vi "Register gRPC Methods.vi"(8 "error in (no error)":errorcluster, 11 "Template Server in":refnum<class "NiDAQmx.lvclass">) -> (0 "error out":errorcluster, 3 "Template Server out":refnum<class "NiDAQmx.lvclass">)   [LabVIEW 2021, in "NI DAQmx_server.lvlib" / "NiDAQmx.lvclass"]
uses:
  NiDAQmx.lvclass
  typeDefs/Server Internal UEs.ctl
  typeDefs/Server Internal Message.ctl
  typeDefs/Server gRPC UEs.ctl
  <vilib>/gRPC/LabVIEW gRPC Library/Server API/typeDefs/gRPCId Cluster.ctl
  <vilib>/gRPC/LabVIEW gRPC Library/Shared/grpcId.ctl
  NiDAQmx.lvclass/NiDAQmx.ctl
  <vilib>/gRPC/LabVIEW gRPC Library/grpc-lvsupport-release.lvlib
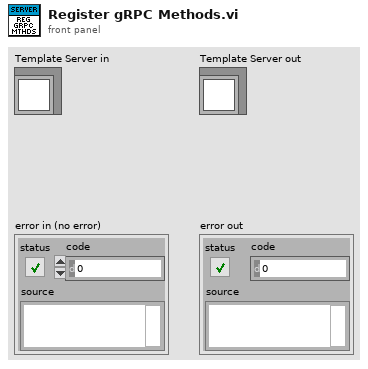
[diagram p1: front panel]
types:
  T1 = typedef "NI DAQmx_server.lvlib/NiDAQmx.lvclass/Server gRPC UEs.ctl" = cluster{"NiDAQmx CreateTask gRPC UE":refnum<user-event>, "NiDAQmx CreateDOChan gRPC UE":refnum<user-event>, "NiDAQmx CreateCIFreqChan gRPC UE":refnum<user-event>, "NiDAQmx WriteDigitalLines gRPC UE":refnum<user-event>, "NiDAQmx ReadCounterScalarF64 gRPC UE":refnum<user-event>, "NiDAQmx CfgImplicitTiming gRPC UE":refnum<user-event>, "NiDAQmx StartTask gRPC UE":refnum<user-event>, "NiDAQmx StopTask gRPC UE":refnum<user-event>, "NiDAQmx ClearTask gRPC UE":refnum<user-event>, "NiDAQmx GetTaskAttributeString gRPC UE":refnum<user-event>, "NiDAQmx GetChanAttributeString gRPC UE":refnum<user-event>, "NiDAQmx GetChanAttributeDouble gRPC UE":refnum<user-event>, "NiDAQmx SetChanAttributeString gRPC UE":refnum<user-event>, "NiDAQmx SetChanAttributeDouble gRPC UE":refnum<user-event>}
  T2 = typedef "NI DAQmx_server.lvlib/NiDAQmx.lvclass/Server Internal UEs.ctl" = cluster{"NiDAQmx CreateTask Internal UE":refnum<user-event>, "NiDAQmx CreateDOChan Internal UE":refnum<user-event>, "NiDAQmx CreateCIFreqChan Internal UE":refnum<user-event>, "NiDAQmx WriteDigitalLines Internal UE":refnum<user-event>, "NiDAQmx ReadCounterScalarF64 Internal UE":refnum<user-event>, "NiDAQmx CfgImplicitTiming Internal UE":refnum<user-event>, "NiDAQmx StartTask Internal UE":refnum<user-event>, "NiDAQmx StopTask Internal UE":refnum<user-event>, "NiDAQmx ClearTask Internal UE":refnum<user-event>, "NiDAQmx GetTaskAttributeString Internal UE":refnum<user-event>, "NiDAQmx GetChanAttributeString Internal UE":refnum<user-event>, "NiDAQmx GetChanAttributeDouble Internal UE":refnum<user-event>, "NiDAQmx SetChanAttributeString Internal UE":refnum<user-event>, "NiDAQmx SetChanAttributeDouble Internal UE":refnum<user-event>}
  T3 = typedef "grpc-lvsupport-release.lvlib/grpcId.ctl" = u64
  T4 = typedef "NI DAQmx_server.lvlib/NiDAQmx.lvclass/Server Internal Message UE.ctl" = refnum<user-event>
  T5 = typedef "grpc-lvsupport-release.lvlib/gRPCId Cluster UE.ctl" = refnum<user-event>
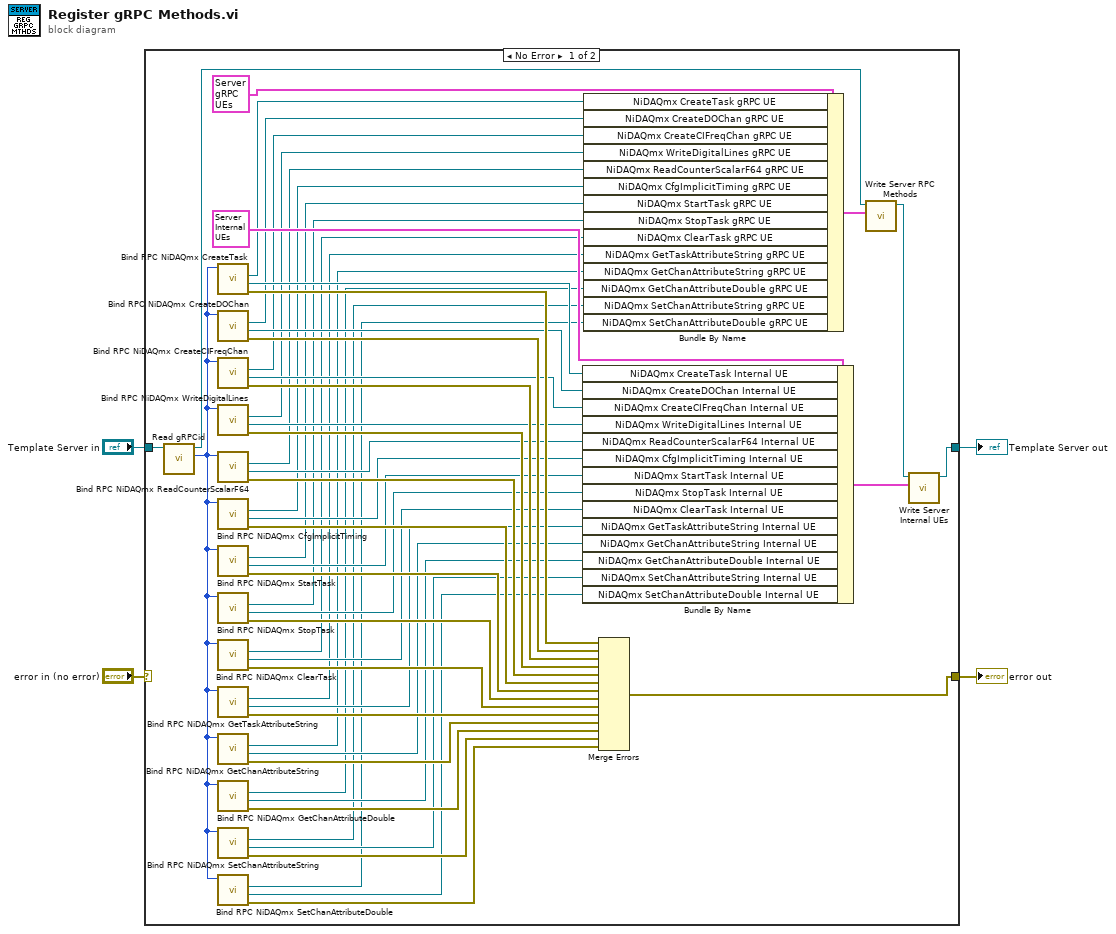
[diagram p0: block diagram]
diagram:
  n1 = case shown="No Error" "error in (no error)" {
    selector: "error in (no error)" -> [_ w57]
    tunnel: "Template Server in" -> [w48 w58]
    tunnel: [w56 w57] -> w3
    tunnel: [w55 w58] -> w2
    frame No Error {
      n2 = call-dynamic "Read gRPCid.vi"("iService in"=w48) -> ("gRPCid"=w47:T3, "iService out"=w49:refnum<class "NiDAQmx.lvclass">)  [unwired: 8 in, 1 out]
      n3 = call "Bind RPC NiDAQmx CreateTask.vi"("gRPCid server in"=w47) -> ("error out"=w46:errorcluster, "NiDAQmx CreateTask Internal UE"=w44:T4, "NiDAQmx CreateTask gRPC UE"=w45:T5)  [unwired: 7 in, 1 out]
      n4 = call "Bind RPC NiDAQmx CreateDOChan.vi"("gRPCid server in"=w47) -> ("error out"=w43:errorcluster, "NiDAQmx CreateDOChan Internal UE"=w41:T4, "NiDAQmx CreateDOChan gRPC UE"=w42:T5)  [unwired: 7 in, 1 out]
      n5 = call "Bind RPC NiDAQmx CreateCIFreqChan.vi"("gRPCid server in"=w47) -> ("error out"=w40:errorcluster, "NiDAQmx CreateCIFreqChan Internal UE"=w38:T4, "NiDAQmx CreateCIFreqChan gRPC UE"=w39:T5)  [unwired: 7 in, 1 out]
      n6 = call "Bind RPC NiDAQmx WriteDigitalLines.vi"("gRPCid server in"=w47) -> ("error out"=w37:errorcluster, "NiDAQmx WriteDigitalLines Internal UE"=w35:T4, "NiDAQmx WriteDigitalLines gRPC UE"=w36:T5)  [unwired: 7 in, 1 out]
      n7 = call "Bind RPC NiDAQmx ReadCounterScalarF64.vi"("gRPCid server in"=w47) -> ("error out"=w34:errorcluster, "NiDAQmx ReadCounterScalarF64 Internal UE"=w32:T4, "NiDAQmx ReadCounterScalarF64 gRPC UE"=w33:T5)  [unwired: 7 in, 1 out]
      n8 = call "Bind RPC NiDAQmx CfgImplicitTiming.vi"("gRPCid server in"=w47) -> ("error out"=w31:errorcluster, "NiDAQmx CfgImplicitTiming Internal UE"=w29:T4, "NiDAQmx CfgImplicitTiming gRPC UE"=w30:T5)  [unwired: 7 in, 1 out]
      n9 = call "Bind RPC NiDAQmx StartTask.vi"("gRPCid server in"=w47) -> ("error out"=w28:errorcluster, "NiDAQmx StartTask Internal UE"=w26:T4, "NiDAQmx StartTask gRPC UE"=w27:T5)  [unwired: 7 in, 1 out]
      n10 = call "Bind RPC NiDAQmx StopTask.vi"("gRPCid server in"=w47) -> ("error out"=w25:errorcluster, "NiDAQmx StopTask Internal UE"=w23:T4, "NiDAQmx StopTask gRPC UE"=w24:T5)  [unwired: 7 in, 1 out]
      n11 = call "Bind RPC NiDAQmx ClearTask.vi"("gRPCid server in"=w47) -> ("error out"=w22:errorcluster, "NiDAQmx ClearTask Internal UE"=w20:T4, "NiDAQmx ClearTask gRPC UE"=w21:T5)  [unwired: 7 in, 1 out]
      n12 = call "Bind RPC NiDAQmx GetTaskAttributeString.vi"("gRPCid server in"=w47) -> ("error out"=w19:errorcluster, "NiDAQmx GetTaskAttributeString Internal UE"=w17:T4, "NiDAQmx GetTaskAttributeString gRPC UE"=w18:T5)  [unwired: 7 in, 1 out]
      n13 = call "Bind RPC NiDAQmx GetChanAttributeString.vi"("gRPCid server in"=w47) -> ("error out"=w16:errorcluster, "NiDAQmx GetChanAttributeString Internal UE"=w14:T4, "NiDAQmx GetChanAttributeString gRPC UE"=w15:T5)  [unwired: 7 in, 1 out]
      n14 = call "Bind RPC NiDAQmx GetChanAttributeDouble.vi"("gRPCid server in"=w47) -> ("error out"=w13:errorcluster, "NiDAQmx GetChanAttributeDouble Internal UE"=w11:T4, "NiDAQmx GetChanAttributeDouble gRPC UE"=w12:T5)  [unwired: 7 in, 1 out]
      n15 = call "Bind RPC NiDAQmx SetChanAttributeString.vi"("gRPCid server in"=w47) -> ("error out"=w10:errorcluster, "NiDAQmx SetChanAttributeString Internal UE"=w8:T4, "NiDAQmx SetChanAttributeString gRPC UE"=w9:T5)  [unwired: 7 in, 1 out]
      n16 = call "Bind RPC NiDAQmx SetChanAttributeDouble.vi"("gRPCid server in"=w47) -> ("error out"=w7:errorcluster, "NiDAQmx SetChanAttributeDouble Internal UE"=w5:T4, "NiDAQmx SetChanAttributeDouble gRPC UE"=w6:T5)  [unwired: 7 in, 1 out]
      n17 = Bundle By Name ("Bundle Internal UEs")(cluster=T2 {"NiDAQmx CreateTask Internal UE"=refnum, "NiDAQmx CreateDOChan Internal UE"=refnum, "NiDAQmx CreateCIFreqChan Internal UE"=refnum, "NiDAQmx WriteDigitalLines Internal UE"=refnum, "NiDAQmx ReadCounterScalarF64 Internal UE"=refnum, "NiDAQmx CfgImplicitTiming Internal UE"=refnum, "NiDAQmx StartTask Internal UE"=refnum, "NiDAQmx StopTask Internal UE"=refnum, "NiDAQmx ClearTask Internal UE"=refnum, "NiDAQmx GetTaskAttributeString Internal UE"=refnum, "NiDAQmx GetChanAttributeString Internal UE"=refnum, "NiDAQmx GetChanAttributeDouble Internal UE"=refnum, "NiDAQmx SetChanAttributeString Internal UE"=refnum, "NiDAQmx SetChanAttributeDouble Internal UE"=refnum} ("Server Internal UEs"), "NiDAQmx CreateTask Internal UE"=w44, "NiDAQmx CreateDOChan Internal UE"=w41, "NiDAQmx CreateCIFreqChan Internal UE"=w38, "NiDAQmx WriteDigitalLines Internal UE"=w35, "NiDAQmx ReadCounterScalarF64 Internal UE"=w32, "NiDAQmx CfgImplicitTiming Internal UE"=w29, "NiDAQmx StartTask Internal UE"=w26, "NiDAQmx StopTask Internal UE"=w23, "NiDAQmx ClearTask Internal UE"=w20, "NiDAQmx GetTaskAttributeString Internal UE"=w17, "NiDAQmx GetChanAttributeString Internal UE"=w14, "NiDAQmx GetChanAttributeDouble Internal UE"=w11, "NiDAQmx SetChanAttributeString Internal UE"=w8, "NiDAQmx SetChanAttributeDouble Internal UE"=w5) -> (w54:T2)
      n18 = Bundle By Name ("Bundle gRPC UEs")(cluster=T1 {"NiDAQmx CreateTask gRPC UE"=refnum, "NiDAQmx CreateDOChan gRPC UE"=refnum, "NiDAQmx CreateCIFreqChan gRPC UE"=refnum, "NiDAQmx WriteDigitalLines gRPC UE"=refnum, "NiDAQmx ReadCounterScalarF64 gRPC UE"=refnum, "NiDAQmx CfgImplicitTiming gRPC UE"=refnum, "NiDAQmx StartTask gRPC UE"=refnum, "NiDAQmx StopTask gRPC UE"=refnum, "NiDAQmx ClearTask gRPC UE"=refnum, "NiDAQmx GetTaskAttributeString gRPC UE"=refnum, "NiDAQmx GetChanAttributeString gRPC UE"=refnum, "NiDAQmx GetChanAttributeDouble gRPC UE"=refnum, "NiDAQmx SetChanAttributeString gRPC UE"=refnum, "NiDAQmx SetChanAttributeDouble gRPC UE"=refnum} ("gRPC Server Method Events"), "NiDAQmx CreateTask gRPC UE"=w45, "NiDAQmx CreateDOChan gRPC UE"=w42, "NiDAQmx CreateCIFreqChan gRPC UE"=w39, "NiDAQmx WriteDigitalLines gRPC UE"=w36, "NiDAQmx ReadCounterScalarF64 gRPC UE"=w33, "NiDAQmx CfgImplicitTiming gRPC UE"=w30, "NiDAQmx StartTask gRPC UE"=w27, "NiDAQmx StopTask gRPC UE"=w24, "NiDAQmx ClearTask gRPC UE"=w21, "NiDAQmx GetTaskAttributeString gRPC UE"=w18, "NiDAQmx GetChanAttributeString gRPC UE"=w15, "NiDAQmx GetChanAttributeDouble gRPC UE"=w12, "NiDAQmx SetChanAttributeString gRPC UE"=w9, "NiDAQmx SetChanAttributeDouble gRPC UE"=w6) -> (w51:T1)
      n19 = Merge Errors(w46, w43, w40, w37, w34, w31, w28, w25, w22, w19, w16, w13, w10, w7) -> (w56:errorcluster)
      n20 = call "Write Server RPC Methods.vi"("Server RPC Methods"=w51, "SignalGeneratorService in"=w49) -> ("SignalGeneratorService out"=w52:refnum<class "NiDAQmx.lvclass">)  [unwired: 8 in, 1 out]
      n21 = call "Write Server Internal UEs.vi"("Server Internal UEs"=w54, "SignalGeneratorService in"=w52) -> ("SignalGeneratorService out"=w55:refnum<class "NiDAQmx.lvclass">)  [unwired: 8 in, 1 out]
    }
    frame Error {
    }
  }
  "error out" <- w3
  "Template Server out" <- w2
